vi "4.4.vi"() -> ()   [LabVIEW 2017]
panel:
  in  "数值":dbl
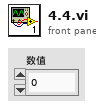
[diagram p1: front panel]
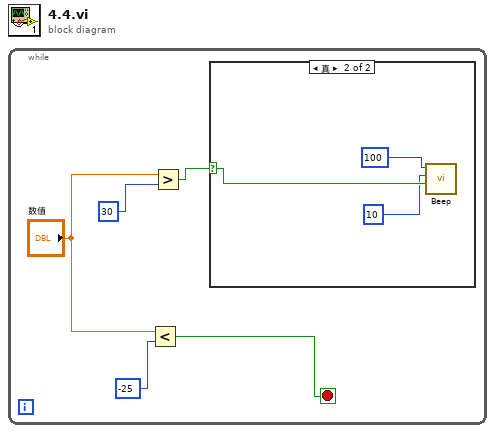
[diagram p0: block diagram]
diagram:
  n1 = while {
    stop <- w2 stop-if-true
    n2 = Less?(x="数值", y=-25) -> (x < y?=w2:bool)
    n3 = Greater?(x="数值", y=30) -> (0:w1:bool)
    n4 = case shown="真" w1 {
      selector: w1 -> [_ w8]
      frame False {
      }
      frame True {
        n5 = call <vilib>:"Beep.vi"("use system alert? (T)"=w8, "duration (msec)"=10, "frequency (Hz)"=100) -> ()  [unwired: 9 in]
      }
    }
  }
